vi "StoreSpecParms.vi"() -> ()   [LabVIEW 2017]
doc: "This example stores and recalls Bias Spectroscopy parameters so it's easy to switch between several spectroscopy configurations.\n\n- Nanonis Programming Interface -"
uses:
  Nanonis Prog Interface.lvlib
panel:
  out "Run after recall":bool
  in  "Settling Time":u32
  out "Amplitude":sgl format="%_5p"
  out "Frequency":dbl format="%_5p"
  out "LockIn":bool
  out "# Points":i32
  out "End":sgl format="%_5p"
  out "Start":sgl format="%_5p"
  out "LI available":bool
  out "ORest&Run":refnum<k4>
  in  "Restore&Run":bool
  out "OUpdateItems":refnum<k4>
  out "ODeleteSelected":refnum<k4>
  in  "Delete Sel":bool
  out "ORestoreSelected":refnum<k4>
  in  "RestoreSelected":bool
  out "OParmsSelected":refnum<k4>
  in  "Params":i32(listbox) caption="Parms"
  out "Parameters":T1(array[cluster])
  out "OGetParms":refnum<k4>
  in  "GetParms":bool
  out "AllQuit":bool
  in  "Quit":bool
  # "Variables"
  # "ms"
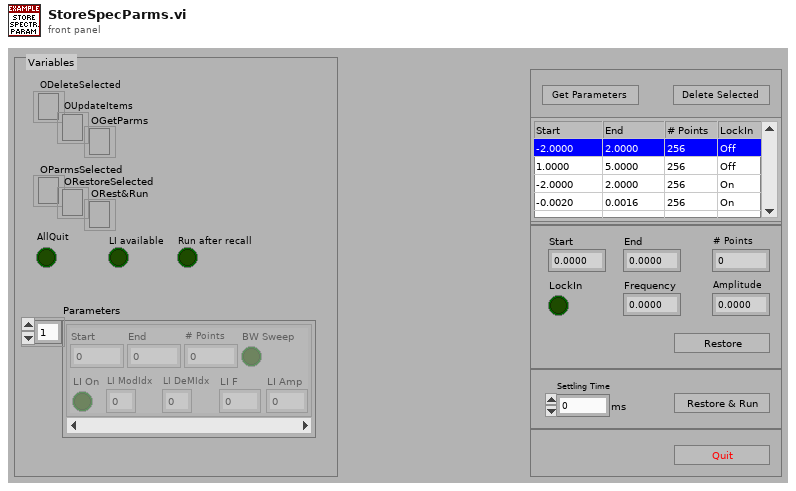
[diagram p1: front panel]
types:
  T1 = cluster{"Start":sgl, "End":sgl, "# Points":i32, "BW Sweep":bool, "LI On":bool, "LI ModIdx":i8, "LI DeMIdx":i8, "LI F":dbl, "LI Amp":sgl}[]
  T2 = cluster{"Start":sgl, "End":sgl, "# Points":i32, "BW Sweep":bool, "LI On":bool, "LI ModIdx":i8, "LI DeMIdx":i8, "LI F":dbl, "LI Amp":sgl}
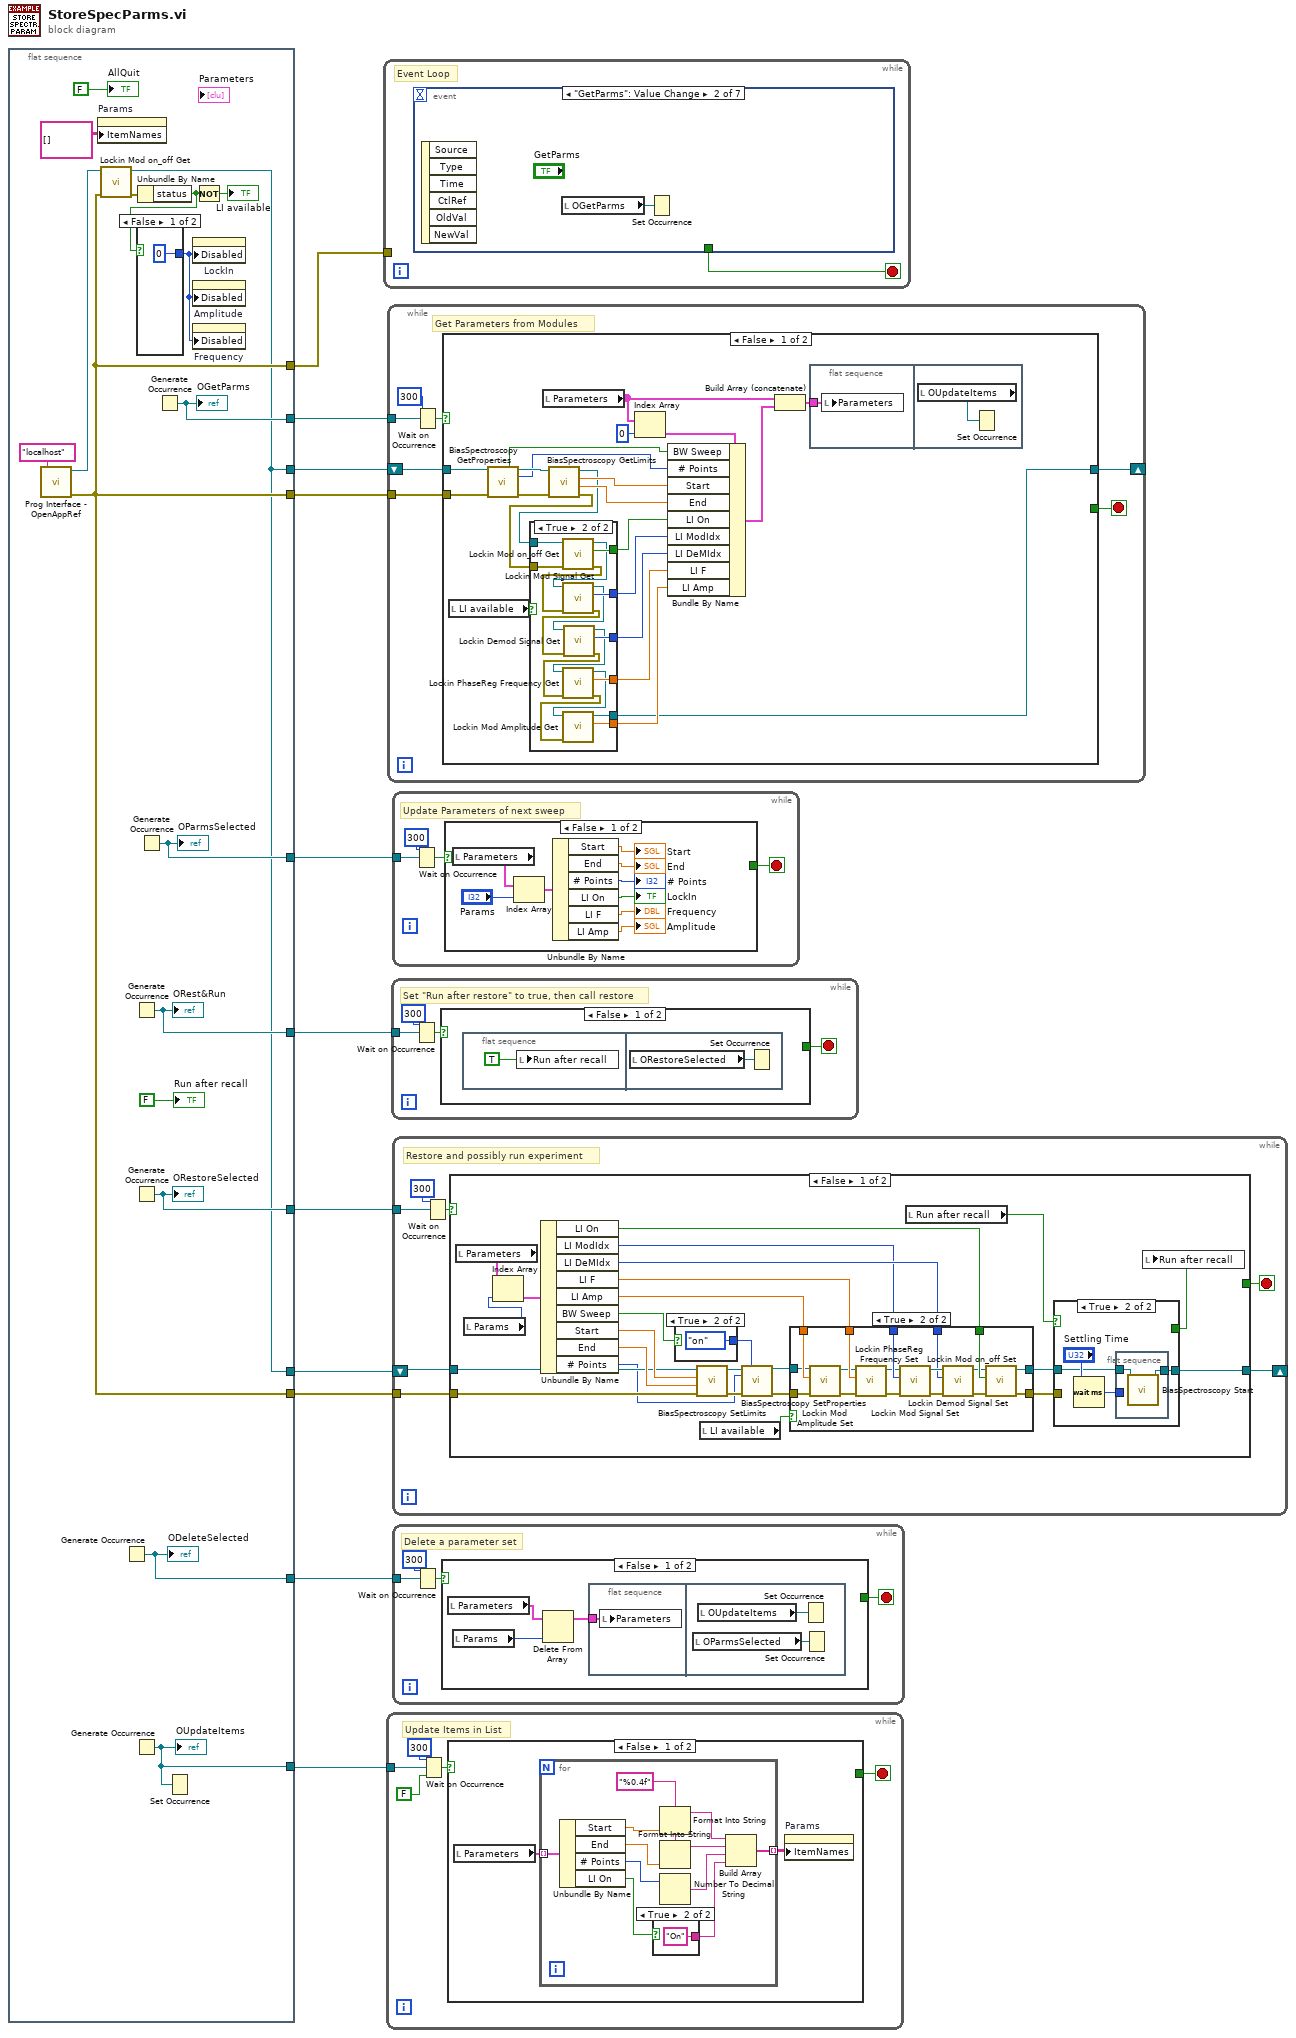
[diagram p0: block diagram]
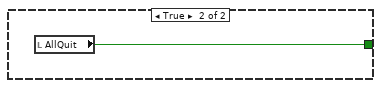
[diagram p2: hidden frame]
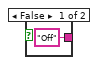
[diagram p3: hidden frame]
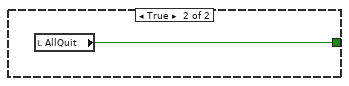
[diagram p4: hidden frame]
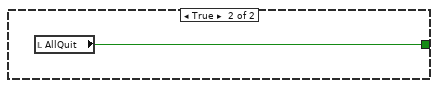
[diagram p5: hidden frame]
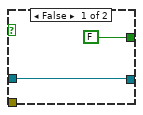
[diagram p7: hidden frame]
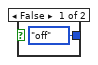
[diagram p8: hidden frame]
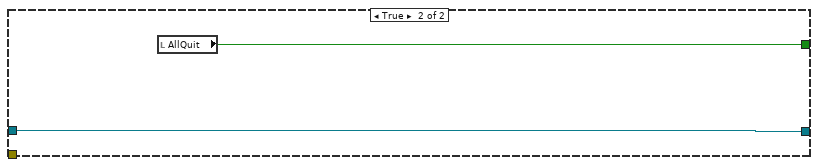
[diagram p9: hidden frame]
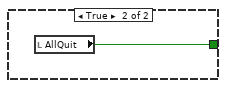
[diagram p10: hidden frame]
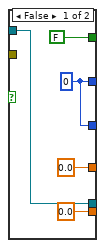
[diagram p11: hidden frame]
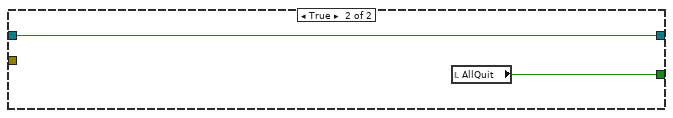
[diagram p12: hidden frame]
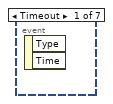
[diagram p13: hidden frame]
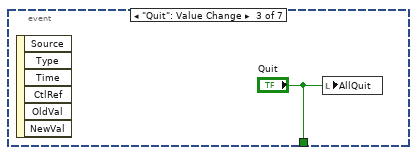
[diagram p14: hidden frame]
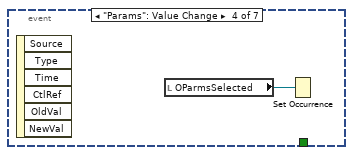
[diagram p15: hidden frame]
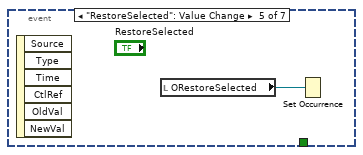
[diagram p16: hidden frame]
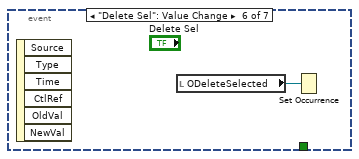
[diagram p17: hidden frame]
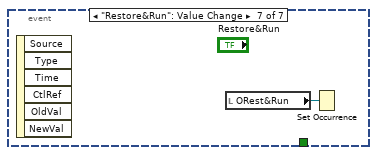
[diagram p18: hidden frame]
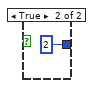
[diagram p19: hidden frame]
diagram:
  n1 = flat-sequence {
    tunnel: [w27] -> w11
    tunnel: [w14] -> w10
    tunnel: [w24] -> w9
    tunnel: [w23] -> w8
    tunnel: [w22] -> w7
    tunnel: [w20] -> w6
    tunnel: [w14] -> w5
    tunnel: [w14] -> w4
    tunnel: [w16] -> w3
    tunnel: [w13] -> w2
    tunnel: [w13] -> w1
    frame #0 {
      n2 = call <userlib>:"Prog Interface - OpenAppRef.vi"("Machine name (local machine IP)"="localhost") -> ("Error out"=w14:errorcluster, "Application reference"=w15:refnum<vi>)  [unwired: 5 in]
      n3 = property on="Params" class="MCListbox (strict)"("ItemNames"=string[][] [] ("Item Names")) -> ()  [unwired: 2 in, 2 out]
      n4 = call <userlib>:"Lockin Mod on_off Get.vi"("Error in (no error)"=w14, "Application ref in"=w15) -> ("Error out"=w12:errorcluster, "Application ref out"=w13:refnum<vi>)  [unwired: 7 in, 1 out]
      n5 = Generate Occurrence() -> (w22:refnum<k4>)
      "ODeleteSelected" <- w22
      n6 = Generate Occurrence() -> (w16:refnum<k4>)
      "ORest&Run" <- w16
      n7 = Generate Occurrence() -> (w23:refnum<k4>)
      "ORestoreSelected" <- w23
      n8 = Generate Occurrence() -> (w20:refnum<k4>)
      "OUpdateItems" <- w20
      n9 = Generate Occurrence() -> (w24:refnum<k4>)
      "OParmsSelected" <- w24
      n10 = Unbundle By Name(w12) -> ("status"=w19:bool)
      n11 = case shown="False" w19 {
        tunnel: [u8 0 ("Disabled") u8 2 ("Disabled")] -> w18
        frame False {
        }
        frame True {
        }
      }
      n12 = Generate Occurrence() -> (w27:refnum<k4>)
      "OGetParms" <- w27
      n13 = Set Occurrence(w20) -> ()
      n14 = property on="LockIn" class="Bool (strict)"("Disabled"=w18) -> ()  [unwired: 2 in, 2 out]
      n15 = property on="Amplitude" class="DigNum (strict)"("Disabled"=w18) -> ()  [unwired: 2 in, 2 out]
      n16 = property on="Frequency" class="DigNum (strict)"("Disabled"=w18) -> ()  [unwired: 2 in, 2 out]
      n17 = Not(x=w19) -> (.not. x?=→"LI available":bool)
      "AllQuit" <- FALSE ("AllQuit")
      "Run after recall" <- FALSE ("Run after recall")
    }
  }
  n18 = while {
    tunnel: w5 -> [_]
    stop <- w31 stop-if-true
    # "Event Loop"
    n19 = event shown="[1] \"GetParms\": Value Change" {
      selector: _ -> [_ _ _ _ _ _ _]
      dyn-events: _ -> [_ _ _ _ _ _ _]
      timeout: _ -> [_ _ _ _ _ _ _]
      tunnel: [_ _ "Quit" _ _ _ _] -> w31
      event Timeout {
        n20 = event-data() -> ()  [unwired: 1 in, 2 out]
      }
      event "GetParms": Value Change {
        n21 = event-data() -> ()  [unwired: 1 in, 6 out]
        n22 = local read "OGetParms"() -> (w32:refnum<k4>)
        n23 = Set Occurrence(w32) -> ()
      }
      event "Quit": Value Change {
        n24 = event-data() -> ()  [unwired: 1 in, 6 out]
        n25 = local write "AllQuit"("Quit") -> ()
      }
      event "Params": Value Change {
        n26 = event-data() -> ()  [unwired: 1 in, 6 out]
        n27 = local read "OParmsSelected"() -> (w34:refnum<k4>)
        n28 = Set Occurrence(w34) -> ()
      }
      event "RestoreSelected": Value Change {
        n29 = event-data() -> ()  [unwired: 1 in, 6 out]
        n30 = local read "ORestoreSelected"() -> (w35:refnum<k4>)
        n31 = Set Occurrence(w35) -> ()
      }
      event "Delete Sel": Value Change {
        n32 = event-data() -> ()  [unwired: 1 in, 6 out]
        n33 = local read "ODeleteSelected"() -> (w36:refnum<k4>)
        n34 = Set Occurrence(w36) -> ()
      }
      event "Restore&Run": Value Change {
        n35 = event-data() -> ()  [unwired: 1 in, 6 out]
        n36 = local read "ORest&Run"() -> (w37:refnum<k4>)
        n37 = Set Occurrence(w37) -> ()
      }
    }
  }
  n38 = while {
    tunnel: w6 -> [w41]
    stop <- w39 stop-if-true
    # "Update Items in List"
    n39 = Wait on Occurrence(1:FALSE ("ignore previous (T)"), 2:w41, 3:300 ("ms timeout (-1)")) -> (0:w40:bool)
    n40 = case shown="False" w40 {
      tunnel: [_ w58] -> w39
      frame False {
        n41 = local read "Parameters"() -> (w44:T1)
        n42 = for {
          tunnel: [w51] -> w43 mode=indexing
          tunnel: w44 -> [w50] mode=indexing
          w45 = "%0.4f" ("format string")
          n43 = Unbundle By Name(w50) -> ("Start"=w49:sgl, "End"=w48:sgl, "# Points"=w55:i32, "LI On"=w54:bool)
          n44 = case shown="True" w54 {
            tunnel: ["Off" "On"] -> w52
            frame False {
            }
            frame True {
            }
          }
          n45 = Format Into String(format string=w45, w49) -> (resulting string=w46:string)  [unwired: 2 in, 1 out]
          n46 = Format Into String(format string=w45, w48) -> (resulting string=w47:string)  [unwired: 2 in, 1 out]
          n47 = Number To Decimal String(number=w55) -> (decimal integer string=w53:string)  [unwired: 1 in]
          n48 = Build Array(w46, w47, w53, w52) -> (w51:string[])
        }
        n49 = property on="Params" class="MCListbox (strict)"("ItemNames"=w43) -> ()  [unwired: 2 in, 2 out]
      }
      frame True {
        n50 = local read "AllQuit"() -> (w58:bool)
      }
    }
  }
  n51 = while {
    tunnel: w11 -> [w65]
    tunnel: w10 -> [w61]
    shift-right: [w59] -> _
    shift-left: w2 -> [w60]
    stop <- w62 stop-if-true
    # "Get Parameters from Modules"
    n52 = Wait on Occurrence(2:w65, 3:300 ("ms timeout (-1)")) -> (0:w63:bool)  [unwired: 1 in]
    n53 = case shown="False" w63 {
      tunnel: [_ w112] -> w62
      tunnel: w61 -> [w84 _]
      tunnel: w60 -> [w72 w111]
      tunnel: [w67 w111] -> w59
      frame False {
        n54 = local read "LI available"() -> (w76:bool)
        n55 = call <userlib>:"BiasSpectroscopy GetProperties.vi"("Application ref in"=w72, "Error in (no error)"=w84) -> ("Backward sweep"=w87:bool, "Application ref out"=w71:refnum<vi>, "Number of points"=w66:i32, "Error out"=w78:errorcluster)  [unwired: 6 in, 4 out]
        n56 = local read "Parameters"() -> (w75:T1)
        n57 = call <userlib>:"BiasSpectroscopy GetLimits.vi"("Error in (no error)"=w78, "Application ref in"=w71) -> ("Error out"=w77:errorcluster, "End value (V)"=w70:sgl, "Start value (V)"=w69:sgl, "Application ref out"=w68:refnum<vi>)  [unwired: 4 in]
        n58 = case shown="True" w76 {
          tunnel: [FALSE w104] -> w83
          tunnel: [w89 w103] -> w82
          tunnel: [w89 w95] -> w81
          tunnel: [sgl 0.0 ("Frequency (Hz)") w101] -> w80
          tunnel: [sgl 0.0 ("Amplitude (mod. signal unit)") w99] -> w79
          tunnel: w77 -> [_ w106]
          tunnel: w68 -> [w88 w105]
          tunnel: [w88 w98] -> w67
          frame False {
            w89 = i8 0 ("Mod. signal index")
          }
          frame True {
            n59 = call <userlib>:"Lockin Mod on_off Get.vi"("Error in (no error)"=w106, "Application ref in"=w105) -> ("Error out"=w108:errorcluster, "Lockin on/off status"=w104:bool, "Application ref out"=w102:refnum<vi>)  [unwired: 7 in]
            n60 = call <userlib>:"Lockin Mod Signal Get.vi"("Error in (no error)"=w108, "Application ref in"=w102) -> ("Error out"=w96:errorcluster, "Mod. signal index"=w103:i32, "Application ref out"=w97:refnum<vi>)  [unwired: 7 in]
            n61 = call <userlib>:"Lockin Demod Signal Get.vi"("Error in (no error)"=w96, "Application ref in"=w97) -> ("Error out"=w93:errorcluster, "Demod. signal index"=w95:i8, "Application ref out"=w94:refnum<vi>)  [unwired: 7 in]
            n62 = call <userlib>:"Lockin PhaseReg Frequency Get.vi"("Error in (no error)"=w93, "Application ref in"=w94) -> ("Error out"=w107:errorcluster, "Frequency (Hz)"=w101:dbl, "Application ref out"=w100:refnum<vi>)  [unwired: 7 in]
            n63 = call <userlib>:"Lockin Mod Amplitude Get.vi"("Error in (no error)"=w107, "Application ref in"=w100) -> ("Amplitude (mod. signal unit)"=w99:sgl, "Application ref out"=w98:refnum<vi>)  [unwired: 7 in, 1 out]
          }
        }
        n64 = Index Array(array=w75, index=0) -> (element=w85:T2)
        n65 = Bundle By Name(cluster=w85, "BW Sweep"=w87, "# Points"=w66, "Start"=w69, "End"=w70, "LI On"=w83, "LI ModIdx"=w82, "LI DeMIdx"=w81, "LI F"=w80, "LI Amp"=w79) -> (w74:T2)
        n66 = Build Array (concatenate)(w75, w74) -> (w73:T1)
        n67 = flat-sequence {
          tunnel: w73 -> [w109]
          frame #0 {
            n68 = local write "Parameters"(w109) -> ()
          }
          frame #1 {
            n69 = local read "OUpdateItems"() -> (w110:refnum<k4>)
            n70 = Set Occurrence(w110) -> ()
          }
        }
      }
      frame True {
        n71 = local read "AllQuit"() -> (w112:bool)
      }
    }
  }
  n72 = while {
    tunnel: w3 -> [w115]
    stop <- w114 stop-if-true
    # "Set \"Run after restore\" to true, then call restore"
    n73 = Wait on Occurrence(2:w115, 3:300 ("ms timeout (-1)")) -> (0:w113:bool)  [unwired: 1 in]
    n74 = case shown="False" w113 {
      tunnel: [_ w119] -> w114
      frame False {
        n75 = flat-sequence {
          frame #0 {
            n76 = local write "Run after recall"(TRUE ("Run after recall")) -> ()
          }
          frame #1 {
            n77 = local read "ORestoreSelected"() -> (w118:refnum<k4>)
            n78 = Set Occurrence(w118) -> ()
          }
        }
      }
      frame True {
        n79 = local read "AllQuit"() -> (w119:bool)
      }
    }
  }
  n80 = while {
    tunnel: w9 -> [w123]
    stop <- w120 stop-if-true
    # "Update Parameters of next sweep"
    n81 = Wait on Occurrence(2:w123, 3:300 ("ms timeout (-1)")) -> (0:w121:bool)  [unwired: 1 in]
    n82 = case shown="False" w121 {
      tunnel: [_ w133] -> w120
      frame False {
        n83 = local read "Parameters"() -> (w132:T1)
        n84 = Index Array(array=w132, index="Params") -> (element=w130:T2)
        n85 = Unbundle By Name(w130) -> ("Start"=→"Start":sgl, "End"=→"End":sgl, "# Points"=→"# Points":i32, "LI On"=→"LockIn":bool, "LI F"=→"Frequency":dbl, "LI Amp"=→"Amplitude":sgl)
      }
      frame True {
        n86 = local read "AllQuit"() -> (w133:bool)
      }
    }
  }
  n87 = while {
    tunnel: w8 -> [w140]
    tunnel: w4 -> [w137]
    shift-right: [w134] -> _
    shift-left: w1 -> [w135]
    stop <- w139 stop-if-true
    # "Restore and possibly run experiment"
    n88 = Wait on Occurrence(2:w140, 3:300 ("ms timeout (-1)")) -> (0:w136:bool)  [unwired: 1 in]
    n89 = case shown="False" w136 {
      tunnel: [_ w196] -> w139
      tunnel: w137 -> [w151 _]
      tunnel: w135 -> [w146 w195]
      tunnel: [w142 w195] -> w134
      frame False {
        n90 = local read "Parameters"() -> (w165:T1)
        n91 = local read "Params"() -> (w164:i32)
        n92 = Index Array(array=w165, index=w164) -> (element=w163:T2)
        n93 = Unbundle By Name(w163) -> ("LI On"=w153:bool, "LI ModIdx"=w154:i8, "LI DeMIdx"=w155:i8, "LI F"=w156:dbl, "LI Amp"=w157:sgl, "BW Sweep"=w152:bool, "Start"=w147:sgl, "End"=w148:sgl, "# Points"=w141:i32)
        n94 = case shown="True" w152 {
          tunnel: [enum16{"no change", "on", "off"}."off" ("Backward sweep (no change)") enum16{"no change", "on", "off"}."on" ("Backward sweep (no change)")] -> w162
          frame False {
          }
          frame True {
          }
        }
        n95 = call <userlib>:"BiasSpectroscopy SetLimits.vi"("Error in (no error)"=w151, "End value (V)"=w148, "Start value (V)"=w147, "Application ref in"=w146) -> ("Error out"=w161:errorcluster, "Application ref out"=w145:refnum<vi>)  [unwired: 4 in]
        n96 = local read "LI available"() -> (w158:bool)
        n97 = call <userlib>:"BiasSpectroscopy SetProperties.vi"("Application ref in"=w145, "Backward sweep (no change)"=w162, "Number of points (0=no change)"=w141, "Error in (no error)"=w161) -> ("Application ref out"=w144:refnum<vi>, "Error out"=w159:errorcluster)  [unwired: 10 in]
        n98 = case shown="True" w158 {
          tunnel: [w167 w182] -> w160
          tunnel: w159 -> [w167 w181]
          tunnel: w157 -> [_ w180]
          tunnel: w156 -> [_ w179]
          tunnel: w155 -> [_ w168]
          tunnel: w154 -> [_ w177]
          tunnel: w153 -> [_ w178]
          tunnel: w144 -> [w166 w176]
          tunnel: [w166 w173] -> w143
          frame False {
          }
          frame True {
            n99 = call <userlib>:"Lockin Mod Amplitude Set.vi"("Error in (no error)"=w181, "Amplitude (mod. signal unit)"=w180, "Application ref in"=w176) -> ("Error out"=w183:errorcluster, "Application ref out"=w175:refnum<vi>)  [unwired: 7 in]
            n100 = call <userlib>:"Lockin PhaseReg Frequency Set.vi"("Error in (no error)"=w183, "Frequency (Hz)"=w179, "Application ref in"=w175) -> ("Error out"=w184:errorcluster, "Application ref out"=w174:refnum<vi>)  [unwired: 7 in]
            n101 = call <userlib>:"Lockin Mod Signal Set.vi"("Error in (no error)"=w184, "Mod. signal index (-1=no change)"=w177, "Application ref in"=w174) -> ("Error out"=w170:errorcluster, "Application ref out"=w172:refnum<vi>)  [unwired: 7 in]
            n102 = call <userlib>:"Lockin Demod Signal Set.vi"("Error in (no error)"=w170, "Demod. signal index (-1=no change)"=w168, "Application ref in"=w172) -> ("Error out"=w169:errorcluster, "Application ref out"=w171:refnum<vi>)  [unwired: 7 in]
            n103 = call <userlib>:"Lockin Mod on_off Set.vi"("Error in (no error)"=w169, "Lockin ON/OFF"=w178, "Application ref in"=w171) -> ("Error out"=w182:errorcluster, "Application ref out"=w173:refnum<vi>)  [unwired: 7 in]
          }
        }
        n104 = local read "Run after recall"() -> (w150:bool)
        n105 = case shown="True" w150 {
          tunnel: w160 -> [_ _]
          tunnel: [FALSE _] -> w149
          tunnel: w143 -> [w185 w188]
          tunnel: [w185 w187] -> w142
          frame False {
          }
          frame True {
            n106 = Wait (ms)(milliseconds to wait="Settling Time") -> (millisecond timer value=w190:u32)
            n107 = flat-sequence {
              tunnel: w190 -> [_]
              tunnel: w188 -> [w192]
              tunnel: [w191] -> w187
              frame #0 {
                n108 = call <userlib>:"BiasSpectroscopy Start.vi"("Application ref in"=w192) -> ("Application ref out"=w191:refnum<vi>)  [unwired: 10 in, 4 out]
              }
            }
          }
        }
        n109 = local write "Run after recall"(w149) -> ()
      }
      frame True {
        n110 = local read "AllQuit"() -> (w196:bool)
      }
    }
  }
  n111 = while {
    tunnel: w7 -> [w199]
    stop <- w198 stop-if-true
    # "Delete a parameter set"
    n112 = Wait on Occurrence(2:w199, 3:300 ("ms timeout (-1)")) -> (0:w197:bool)  [unwired: 1 in]
    n113 = case shown="False" w197 {
      tunnel: [_ w207] -> w198
      frame False {
        n114 = local read "Parameters"() -> (w203:T1)
        n115 = local read "Params"() -> (w202:i32)
        n116 = Delete From Array(array=w203, index=w202) -> (array with subset deleted=w201:T1)  [unwired: 1 in, 1 out]
        n117 = flat-sequence {
          tunnel: w201 -> [w204]
          frame #0 {
            n118 = local write "Parameters"(w204) -> ()
          }
          frame #1 {
            n119 = local read "OParmsSelected"() -> (w205:refnum<k4>)
            n120 = local read "OUpdateItems"() -> (w206:refnum<k4>)
            n121 = Set Occurrence(w206) -> ()
            n122 = Set Occurrence(w205) -> ()
          }
        }
      }
      frame True {
        n123 = local read "AllQuit"() -> (w207:bool)
      }
    }
  }
